vi "Get Channel.vi"(8 "error in (no error)":errorcluster, 10 "Channel Name":string, 11 "CIFCorePlugin in":refnum<class "CIFCorePlugin.lvclass">) -> (0 "error out":errorcluster, 2 "Channel":refnum<class "CIFChannels.lvclass">, 3 "CIFCorePlugin out":refnum<class "CIFCorePlugin.lvclass">)   [LabVIEW 2021, in "CIFCorePlugin.lvclass"]
uses:
  CIFCorePlugin.lvclass
  CIFUtilities/CIFChannels/CIFChannels.lvclass
  CIFCorePlugin.lvclass/CIFCorePlugin.ctl
  CIFUtilities/CIFChannelMng/CIFChannelMng.lvclass/CIFChannelMng.ctl
  CIFUtilities/CIFClocks/SubVIs/Add Error.vi
  Common/Utilities/Append Error Location.vi
  CIFUtilities/CIFChannelMng/CIFChannelMng.lvclass
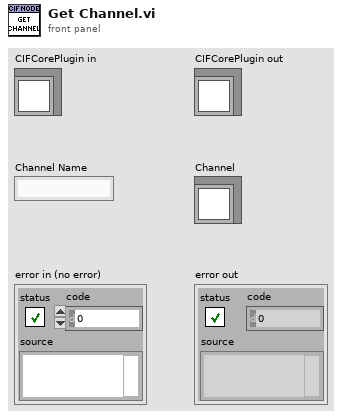
[diagram p1: front panel]
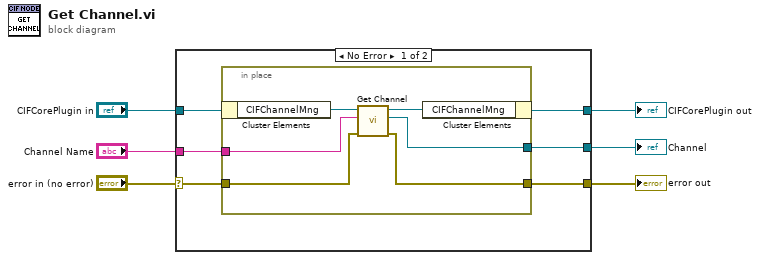
[diagram p0: block diagram]
diagram:
  n1 = case shown="No Error" "error in (no error)" {
    selector: "error in (no error)" -> [w8 w20]
    tunnel: [w7 w20] -> w5
    tunnel: [w11 w19] -> w3
    tunnel: "CIFCorePlugin in" -> [w12 w19]
    tunnel: "Channel Name" -> [w10 _]
    tunnel: [w9 _] -> w1
    frame No Error {
      n2 = in-place {
        in-place-border: w10 -> [w16]
        in-place-border: [w15] -> w9
        in-place-border: w8 -> [w14]
        in-place-border: [w13] -> w7
        n3 = in-place-cluster #1(w12) -> ("CIFChannelMng"=w18:refnum<class "CIFChannelMng.lvclass">)
        n4 = call "Get Channel.vi"("error in (no error)"=w14, "Channel Name"=w16, "CIFChannelMng in"=w18) -> ("error out"=w13:errorcluster, "Channel"=w15:refnum<class "CIFChannels.lvclass">, "CIFChannelMng out"=w17:refnum<class "CIFChannelMng.lvclass">)  [unwired: 6 in]
        n5 = in-place-cluster #1("CIFChannelMng"=w17) -> (w11:refnum<class "CIFCorePlugin.lvclass">)
      }
    }
    frame Error {
    }
  }
  "error out" <- w5
  "CIFCorePlugin out" <- w3
  "Channel" <- w1
